vi "GObject Target String.vi"(11 "GObject":refnum<vi>) -> (3 "Target":string)   [LabVIEW 2016, in "Better Search.lvlib" / "Search Result.lvclass"]
uses:
  Search Result.lvclass
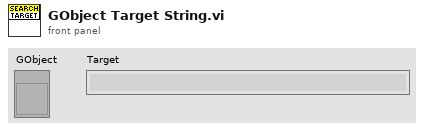
[diagram p1: front panel]
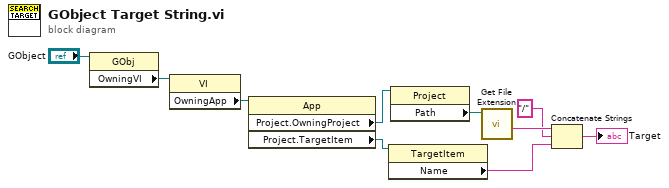
[diagram p0: block diagram]
diagram:
  n1 = property class="GObj"(reference="GObject") -> ("OwningVI"=w9:refnum<vi>)  [unwired: 1 in, 2 out]
  n2 = property class="VI"(reference=w9) -> ("OwningApp"=w8:refnum<vi>)  [unwired: 1 in, 2 out]
  n3 = property class="App"(reference=w8) -> ("Project.OwningProject"=w7:refnum<vi>, "Project.TargetItem"=w5:refnum<vi>)  [unwired: 1 in, 2 out]
  n4 = property class="TargetItem"(reference=w5) -> ("Name"=w3:string)  [unwired: 1 in, 2 out]
  n5 = property class="Project"(reference=w7) -> ("Path"=w6:path)  [unwired: 1 in, 2 out]
  n6 = call <vilib>:"Get File Extension.vi"("file"=w6) -> ("filename without extension"=w4:string)  [unwired: 6 in, 4 out]
  n7 = Concatenate Strings(w4, "/" ("string"), w3) -> (→"Target":string)
